vi "Actuonix LAX breaker actuator subVI.vi"(8 "error in (no error)":errorcluster, 10 "actionEnum":enum16{"OFF", "ON", "RESET"}(ring), 11 "Digital in":refnum<vi>) -> (0 "error out":errorcluster, 2 "position":dbl, 3 "Breaker State":bool)   [LabVIEW 2019]
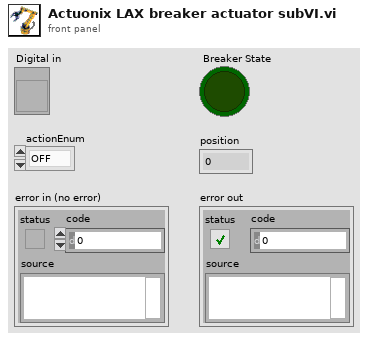
[diagram p1: front panel]
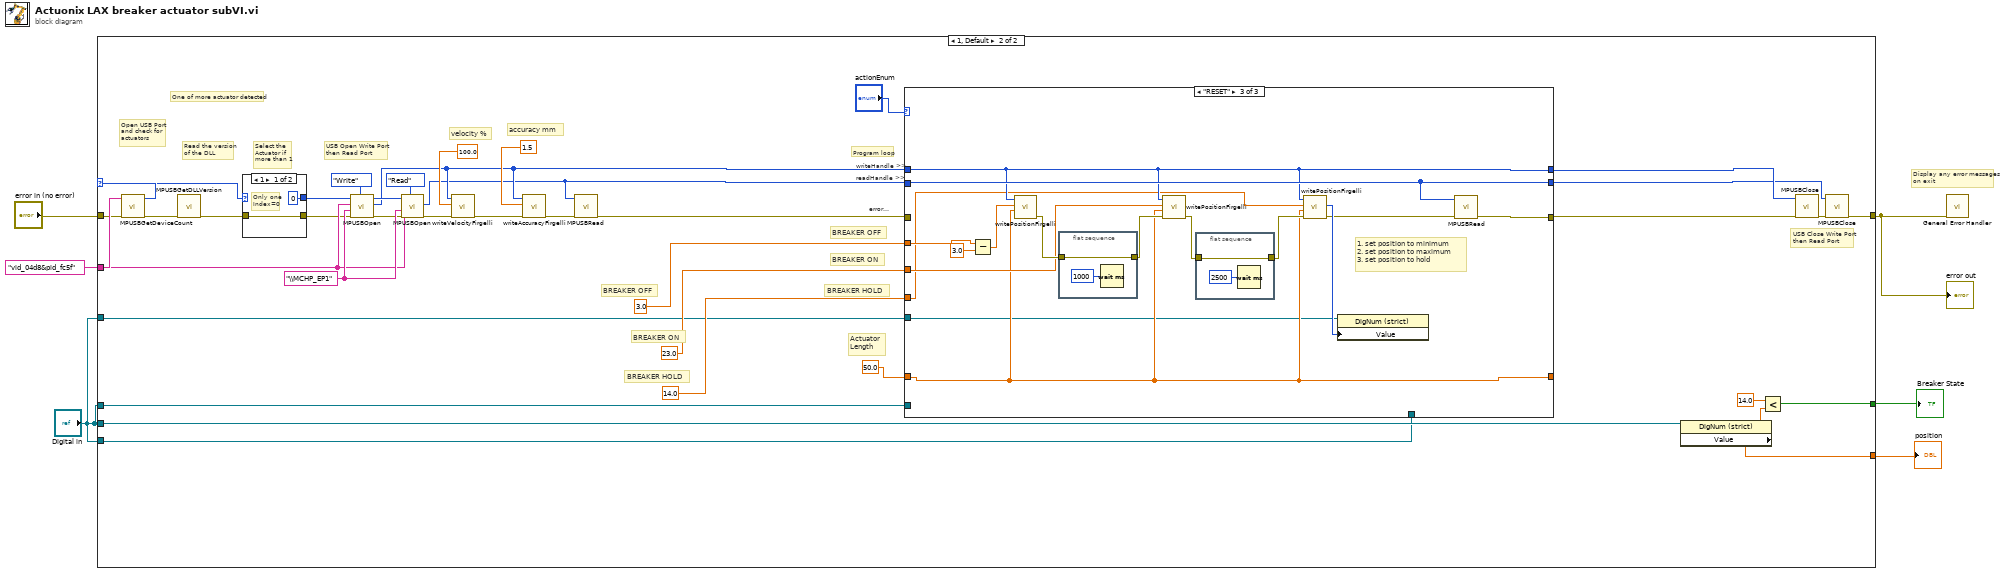
[diagram p0: block diagram]
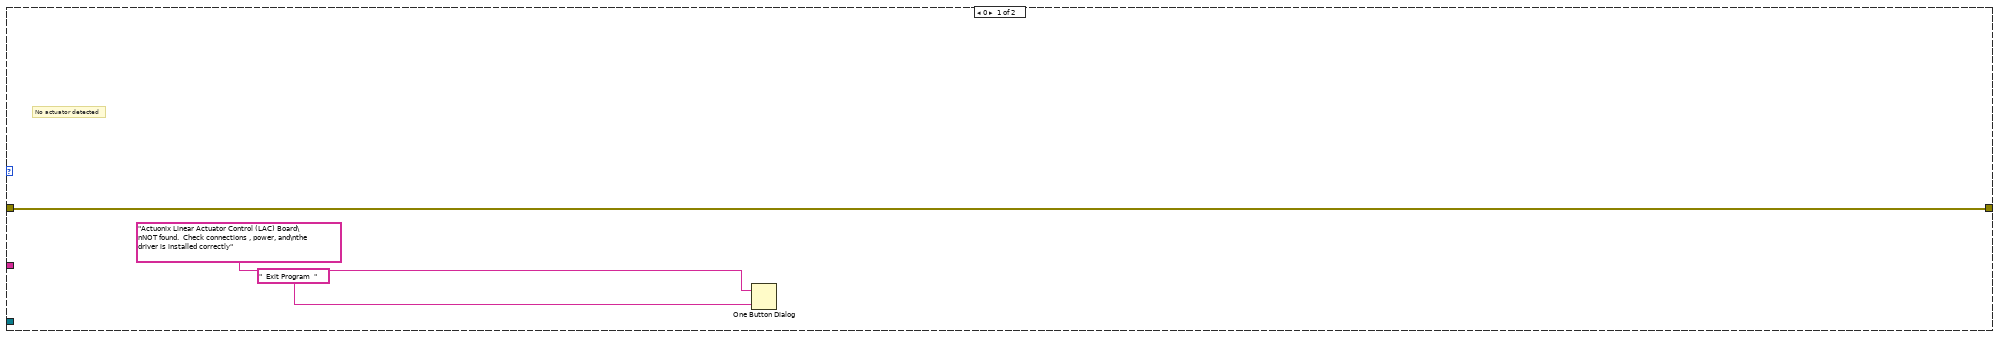
[diagram p2: hidden frame]
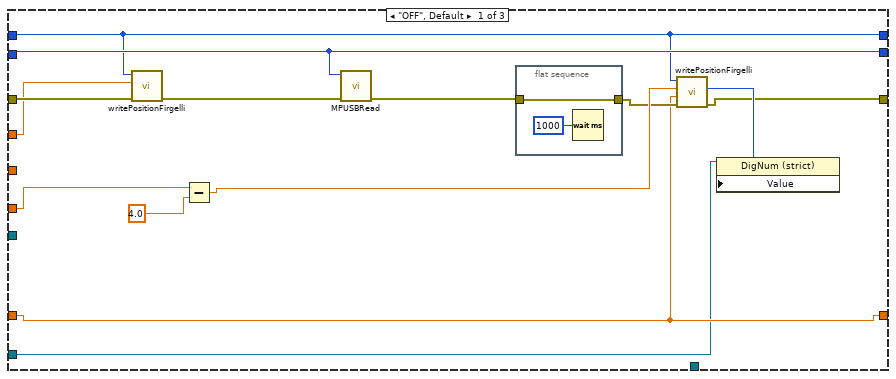
[diagram p3: hidden frame]
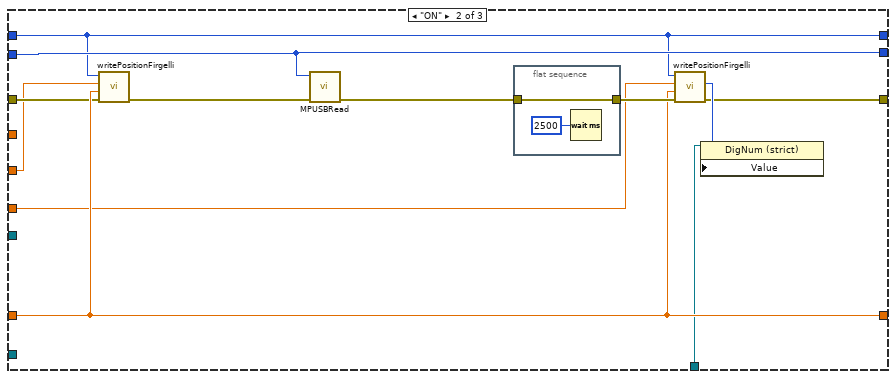
[diagram p4: hidden frame]
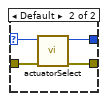
[diagram p5: hidden frame]
diagram:
  w2 = "vid_04d8&pid_fc5f"
  # "Display any error messages\non exit"
  n1 = call "MPUSBGetDeviceCount.vi"("pVID_PID"=w2) -> ("return_value"=w3:u32)  [unwired: 1 in, 9 out]
  n2 = case shown="1, Default" w3 {
    selector: w3 -> [_ w35]
    tunnel: [w8 w41] -> w4
    tunnel: w2 -> [_ w40]
    tunnel: "error in (no error)" -> [w8 w20]
    tunnel: [_ w19] -> w6
    tunnel: [_ w18] -> w7
    tunnel: "Digital in" -> [_ w14]
    tunnel: "Digital in" -> [_ w13]
    tunnel: "Digital in" -> [_ w12]
    tunnel: "Digital in" -> [_ w11]
    frame 0 {
      # "No actuator detected"
      n3 = One Button Dialog(message="Actuonix Linear Actuator Control (LAC) Board\nNOT found.  Check connections , power, and\nthe driver is installed correctly", button name ("OK")="  Exit Program  ") -> ()  [unwired: 1 out]
    }
    frame 1, Default {
      w46 = "\\MCHP_EP1" ("pEP")
      # "BREAKER HOLD"
      # "BREAKER ON"
      # "BREAKER OFF"
      # "Open USB Port\nand check for\nactuators"
      # "Actuator\nLength"
      # "BREAKER HOLD"
      # "BREAKER ON"
      # "BREAKER OFF"
      # "Program loop"
      # "error >>"
      # "readHandle >>"
      # "writeHandle >>"
      # "accuracy mm"
      # "velocity %"
      # "One of more actuator detected"
      # "Select the\nActuator if\nmore than 1"
      # "Read the version\nof the DLL"
      # "USB Open Write Port\nthen Read Port"
      # "USB Close Write Port\nthen Read Port"
      n4 = call "MPUSBGetDLLVersion.vi"("error in (no error)"=w20) -> ("error out"=w39:errorcluster)  [unwired: 10 out]
      n5 = case shown="1" w35 {
        selector: w35 -> [_ w99]
        tunnel: w39 -> [w98 w102]
        tunnel: [w98 w101] -> w38
        tunnel: [u32 0 ("Selected") w100] -> w37
        frame 1 {
          # "Only one\nIndex=0"
        }
        frame Default {
          n6 = call "actuatorSelect.vi"("error in (no error)"=w102, "Devices"=w99) -> ("error out"=w101:errorcluster, "Selected"=w100:u32)  [unwired: 8 out]
        }
      }
      n7 = call "MPUSBOpen.vi"("dwDir"=enum16{"Write", "Read"}."Write", "error in (no error)"=w38, "pEP"=w46, "pVID_PID"=w40, "instance"=w37) -> ("error out"=w43:errorcluster, "HANDLE"=w26:u32, "instanceOut"=w36:u32)  [unwired: 4 in]
      n8 = call "MPUSBOpen.vi"("dwDir"=enum16{"Write", "Read"}."Read", "error in (no error)"=w43, "pEP"=w46, "pVID_PID"=w40, "instance"=w36) -> ("error out"=w33:errorcluster, "HANDLE"=w25:u32)  [unwired: 3 in, 2 out]
      n9 = call "writeVelocityFirgelli.vi"("error in (no error)"=w33, "Velocity"=100.0 ("Velocity (%)"), "handleIn"=w26) -> ("error out"=w31:errorcluster)  [unwired: 8 out]
      n10 = call "writeAccuracyFirgelli.vi"("error in (no error)"=w31, "accuracy"=1.5 ("Accuracy (mm)"), "handleIn"=w26) -> ("error out"=w30:errorcluster)  [unwired: 1 in, 7 out]
      n11 = call "MPUSBRead.vi"("error in (no error)"=w30, "handleIn"=w25) -> ("error out"=w24:errorcluster)  [unwired: 4 in, 5 out]
      n12 = case shown="\"RESET\"" "actionEnum" {
        tunnel: [w50 w66 w82] -> w23
        tunnel: [w51 w67 w83] -> w22
        tunnel: [w52 w70 w84] -> w21
        tunnel: [w53 w69 w78] -> _
        tunnel: 50.0 ("length") -> [w53 w69 w78]
        tunnel: w24 -> [w54 w68 _]
        tunnel: w25 -> [w51 w67 w83]
        tunnel: w26 -> [w50 w66 w82]
        tunnel: 3.0 -> [w48 _ w81]
        tunnel: 23.0 -> [_ w65 w80]
        tunnel: 14.0 -> [w49 w64 w79]
        tunnel: w13 -> [w47 _ _]
        tunnel: w12 -> [_ w63 _]
        tunnel: w11 -> [_ _ w77]
        frame "OFF", Default {
          n13 = call "writePositionFirgelli.vi"("error in (no error)"=w54, "Position (mm)"=w48, "handleIn"=w50) -> ("error out"=w55:errorcluster)  [unwired: 1 in, 7 out]
          n14 = Subtract(x=w49, y=4.0 ("x")) -> (x-y=w59:dbl)
          n15 = call "MPUSBRead.vi"("error in (no error)"=w55, "handleIn"=w51) -> ("error out"=w56:errorcluster)  [unwired: 4 in, 5 out]
          n16 = flat-sequence {
            tunnel: w56 -> [w61]
            tunnel: [w61] -> w57
            frame #0 {
              n17 = Wait (ms)(milliseconds to wait=u32 1000) -> ()  [unwired: 1 out]
            }
          }
          n18 = call "writePositionFirgelli.vi"("error in (no error)"=w57, "lengthMax"=w53, "Position (mm)"=w59, "handleIn"=w50) -> ("error out"=w52:errorcluster, "regSetting"=w60:u16)  [unwired: 6 out]
          n19 = property on="Property Node" class="DigNum (strict)"(reference=w47, "Value"=w60) -> ()  [unwired: 1 in, 2 out]
        }
        frame "ON" {
          n20 = call "writePositionFirgelli.vi"("error in (no error)"=w68, "lengthMax"=w69, "Position (mm)"=w65, "handleIn"=w66) -> ("error out"=w71:errorcluster)  [unwired: 7 out]
          n21 = call "MPUSBRead.vi"("error in (no error)"=w71, "handleIn"=w67) -> ("error out"=w72:errorcluster)  [unwired: 4 in, 5 out]
          n22 = flat-sequence {
            tunnel: w72 -> [w75]
            tunnel: [w75] -> w73
            frame #0 {
              n23 = Wait (ms)(milliseconds to wait=u32 2500) -> ()  [unwired: 1 out]
            }
          }
          n24 = call "writePositionFirgelli.vi"("error in (no error)"=w73, "lengthMax"=w69, "Position (mm)"=w64, "handleIn"=w66) -> ("error out"=w70:errorcluster, "regSetting"=w74:u16)  [unwired: 6 out]
          n25 = property on="Property Node" class="DigNum (strict)"(reference=w63, "Value"=w74) -> ()  [unwired: 1 in, 2 out]
        }
        frame "RESET" {
          # "1. set position to minimum\n2. set position to maximum \n3. set position to hold"
          n26 = Subtract(x=w81, y=3.0) -> (x-y=w91:dbl)
          n27 = call "writePositionFirgelli.vi"("lengthMax"=w78, "Position (mm)"=w91, "handleIn"=w82) -> ("error out"=w86:errorcluster)  [unwired: 1 in, 7 out]
          n28 = flat-sequence {
            tunnel: w86 -> [w95]
            tunnel: [w95] -> w87
            frame #0 {
              n29 = Wait (ms)(milliseconds to wait=u32 1000) -> ()  [unwired: 1 out]
            }
          }
          n30 = call "writePositionFirgelli.vi"("error in (no error)"=w87, "lengthMax"=w78, "Position (mm)"=w80, "handleIn"=w82) -> ("error out"=w88:errorcluster)  [unwired: 7 out]
          n31 = flat-sequence {
            tunnel: w88 -> [w93]
            tunnel: [w93] -> w89
            frame #0 {
              n32 = Wait (ms)(milliseconds to wait=u32 2500) -> ()  [unwired: 1 out]
            }
          }
          n33 = call "writePositionFirgelli.vi"("error in (no error)"=w89, "lengthMax"=w78, "Position (mm)"=w79, "handleIn"=w82) -> ("error out"=w85:errorcluster, "regSetting"=w90:u16)  [unwired: 6 out]
          n34 = property on="Property Node" class="DigNum (strict)"(reference=w77, "Value"=w90) -> ()  [unwired: 1 in, 2 out]
          n35 = call "MPUSBRead.vi"("error in (no error)"=w85, "handleIn"=w83) -> ("error out"=w84:errorcluster)  [unwired: 4 in, 5 out]
        }
      }
      n36 = property on="Property Node" class="DigNum (strict)"(reference=w14) -> ("Value"=w18:dbl)  [unwired: 1 in, 2 out]
      n37 = Less?(x=14.0, y=w18) -> (x < y?=w19:bool)
      n38 = call "MPUSBClose.vi"("error in (no error)"=w21, "handle"=w23) -> ("error out"=w42:errorcluster)  [unwired: 1 in, 8 out]
      n39 = call "MPUSBClose.vi"("error in (no error)"=w42, "handle"=w22) -> ("error out"=w41:errorcluster)  [unwired: 1 in, 8 out]
    }
  }
  "error out" <- w4
  "Breaker State" <- w6
  "position" <- w7
  n40 = call <vilib>:"General Error Handler.vi"("error in (no error)"=w4) -> ()  [unwired: 2 in, 13 out]
